vi "MultiChannel Butterworth Filter PtByPt.vi"(5 "initialize":bool, 6 "order":i32=2, 7 "filter type":T1, 8 "low cutoff freq: fl":dbl=0.125 format="%0.3f", 9 "high cutoff freq: fh":dbl=0.45000000000000007 format="%0.3f", 10 "sampling freq: fs":dbl=1.0 format="%0.2f", 11 "x":dbl[](array[numeric])) -> (0 "error":i32, 3 "Filtered x":dbl[](array[numeric]))   [LabVIEW 2011, in "Filter VIs.lvlib"]
uses:
  Filter VIs.lvlib
  <vilib>/Analysis/3filter.llb/Filter Passband Type.ctl
  <vilib>/Analysis/NI_AALBase.lvlib
panel:
  out "error 2":i32[](array[numeric])
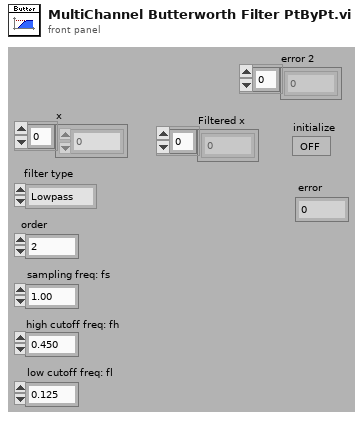
[diagram p1: front panel]
types:
  T1 = typedef "NI_AALBase.lvlib/Filter Passband Type.ctl" = enum32{"Lowpass", "Highpass", "Bandpass", "Bandstop"}
  T2 = cluster{"filter structure":enum32{"IIR 2nd Order", "IIR 4th Order"}, "Reverse Coefficients":dbl[], "Forward Coefficients":dbl[]}
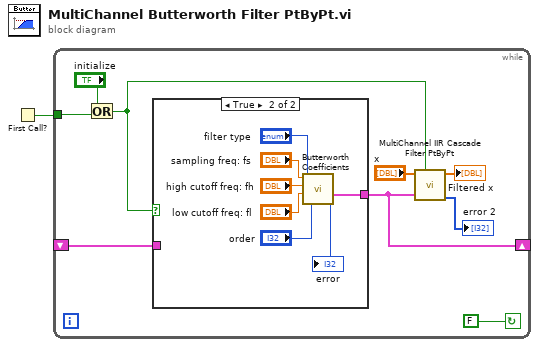
[diagram p0: block diagram]
diagram:
  n1 = First Call?() -> (First Call?: T/F=w1:bool)
  n2 = while {
    tunnel: w1 -> [w6]
    shift-left: _ -> [w9]
    shift-right: [w10] -> _
    stop <- FALSE continue-if-true
    n3 = Or(x="initialize", y=w6) -> (x .or. y?=w5:bool)
    n4 = case shown="True" w5 {
      tunnel: [w11 w14] -> w10
      tunnel: w9 -> [w11 _]
      frame False {
      }
      frame True {
        n5 = call <vilib>:"Butterworth Coefficients.vi"("order"="order", "filter type"="filter type", "low cutoff freq: fl"="low cutoff freq: fl", "high cutoff freq: fh"="high cutoff freq: fh", "sampling freq: fs"="sampling freq: fs") -> ("error"=→"error":i32, "IIR Filter Cluster"=w14:T2)  [unwired: 5 in]
      }
    }
    n6 = call "MultiChannel IIR Cascade Filter PtByPt.vi"("initialize"=w5, "IIR Filter Cluster"=w10, "x"="x") -> ("error"=→"error 2":i32[], "Filtered x"=→"Filtered x":dbl[])  [unwired: 7 in]
  }
